vi "Set ParentNode Selected.vi"(7 "Tri-State?":bool=TRUE, 8 "error in (no error)":errorcluster, 9 "Symbol Index":i32, 10 "Tag":string, 11 "TreeControl in":refnum<vi>) -> (0 "error out":errorcluster, 2 "Seted Tags":T1(array[cluster]), 3 "TreeControl out":refnum<vi>)   [LabVIEW 2023, in "DSLV_Tree.lvlib"]
uses:
  DSLV_Tree.lvlib
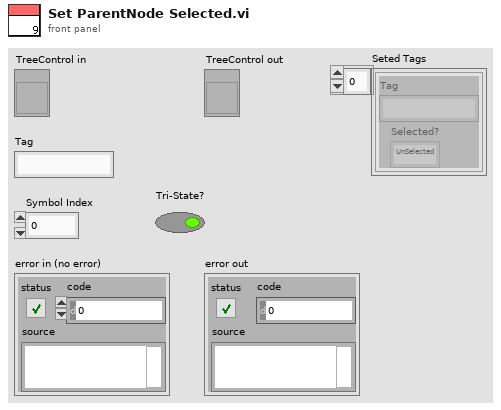
[diagram p1: front panel]
types:
  T1 = cluster{"Tag":string, "Selected?":enum16{"UnSelected", "Selected", "PartSelected"}}[]
  T2 = cluster{"Tag":string, "Selected?":enum16{"UnSelected", "Selected", "PartSelected"}}
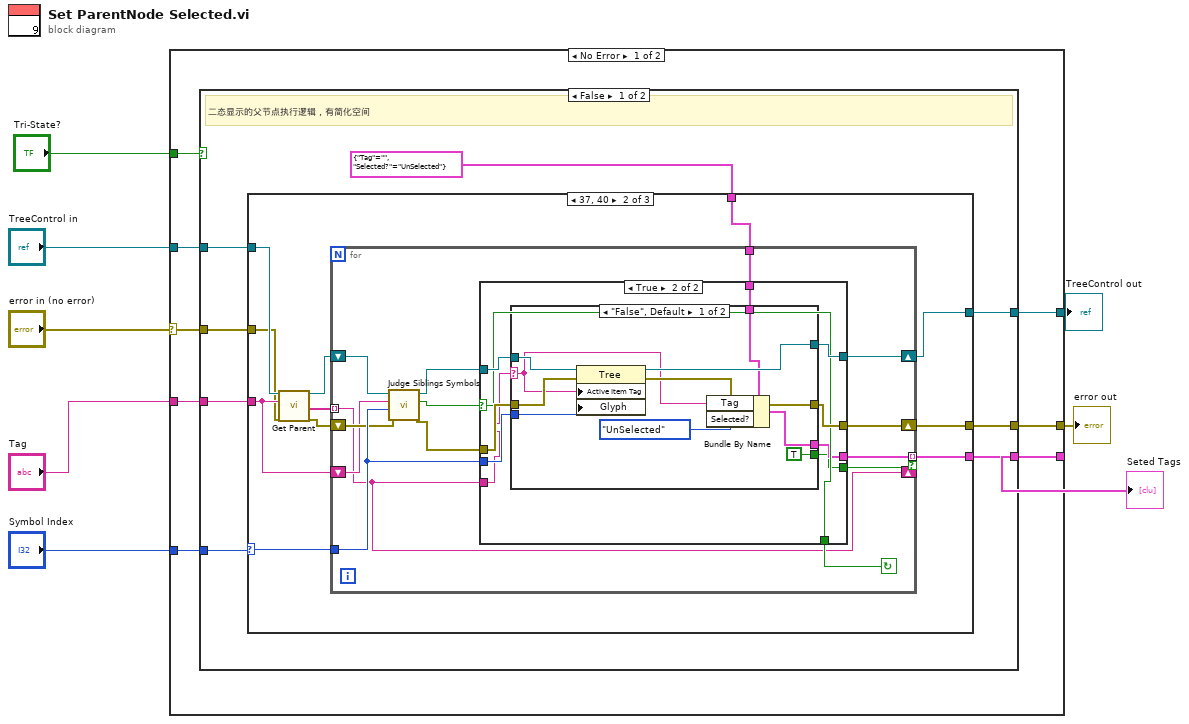
[diagram p0: block diagram]
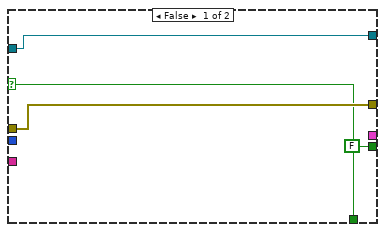
[diagram p3: hidden frame]
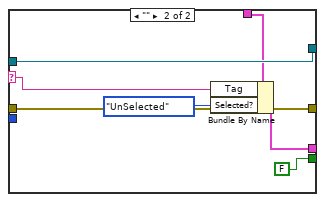
[diagram p4: hidden frame]
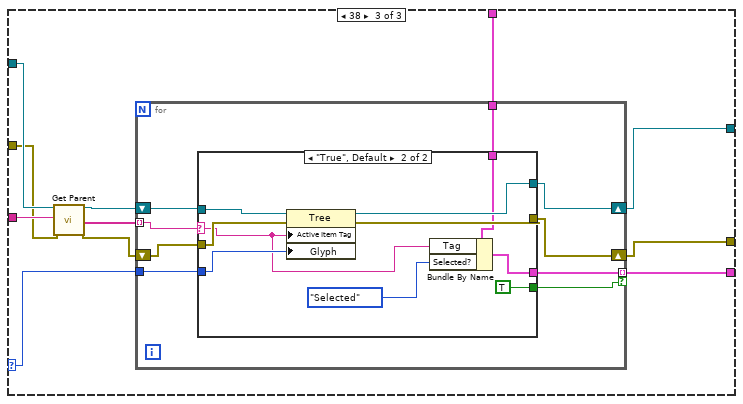
[diagram p5: hidden frame]
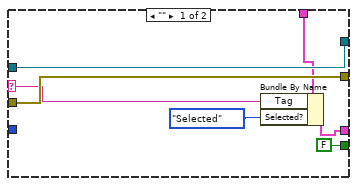
[diagram p6: hidden frame]
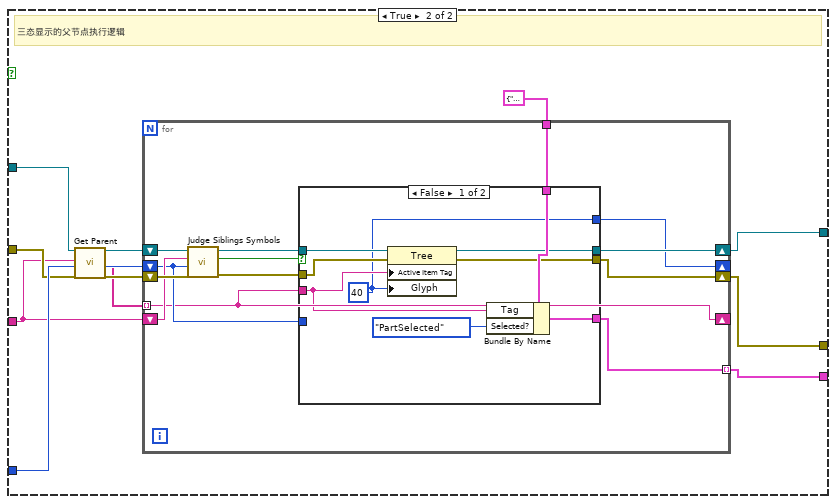
[diagram p7: hidden frame]
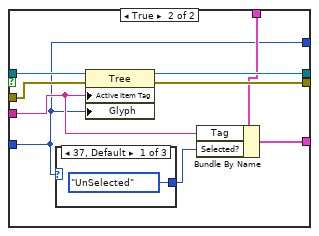
[diagram p8: hidden frame]
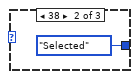
[diagram p9: hidden frame]
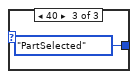
[diagram p10: hidden frame]
diagram:
  n1 = case shown="No Error" "error in (no error)" {
    selector: "error in (no error)" -> [w11 w165]
    tunnel: [w16 w165] -> w8
    tunnel: "Tag" -> [w15 _]
    tunnel: [w14 w166] -> w6
    tunnel: "TreeControl in" -> [w13 w166]
    tunnel: "Symbol Index" -> [w12 _]
    tunnel: [w10 _] -> w2
    tunnel: "Tri-State?" -> [w9 _]
    frame No Error {
      n2 = case shown="False" w9 {
        tunnel: [w24 w120] -> w16
        tunnel: w15 -> [w23 w126]
        tunnel: [w22 w121] -> w14
        tunnel: w13 -> [w21 w129]
        tunnel: w12 -> [w20 w130]
        tunnel: w11 -> [w19 w128]
        tunnel: [w18 w122] -> w10
        frame False {
          # "二态显示的父节点执行逻辑，有简化空间"
          n3 = case shown="37, 40" w20 {
            selector: w20 -> [_ w35 w87]
            tunnel: [w25 w37 w85] -> w24
            tunnel: w23 -> [_ w31 w92]
            tunnel: [w26 w36 w89] -> w22
            tunnel: w19 -> [w25 w30 w86]
            tunnel: w21 -> [w26 w33 w93]
            tunnel: [_ w34 w84] -> w18
            tunnel: T2 {"Tag"="", "Selected?"=enum."UnSelected"} ("Set") -> [_ w27 w83]
            frame -1, Default {
            }
            frame 37, 40 {
              n4 = call "Get Parent.vi"("Tree Reference In"=w33, "Child Tag (Current)"=w31, "error in (no error)"=w30) -> ("Tree Reference Out"=w32:refnum<vi>, "Parents Tags"=w28:string[], "error out"=w29:errorcluster)  [unwired: 13 in, 1 out]
              n5 = for {
                tunnel: w35 -> [w46]
                tunnel: [w45] -> w34 mode=indexing if=w40
                shift-right: [w50] -> w36
                shift-left: w32 -> [w44]
                shift-right: [w51] -> w37
                shift-left: w29 -> [w43]
                tunnel: w28 -> [w38] mode=indexing
                tunnel: w27 -> [w41]
                shift-right: [w38] -> _
                shift-left: w31 -> [w39]
                stop <- w42 continue-if-true
                n6 = call "Judge Siblings Symbols.vi"("error in (no error)"=w43, "Symbol"=w46, "Tag"=w39, "TreeControl in"=w44) -> ("error out"=w48:errorcluster, "The Same?"=w47:bool, "TreeControl out"=w49:refnum<vi>)  [unwired: 5 in]
                n7 = case shown="True" w47 {
                  selector: w47 -> [w53 w59]
                  tunnel: w48 -> [w54 w62]
                  tunnel: w49 -> [w55 w65]
                  tunnel: [w55 w64] -> w50
                  tunnel: [w54 w63] -> w51
                  tunnel: w46 -> [_ w61]
                  tunnel: [_ w57] -> w45
                  tunnel: w38 -> [_ w60]
                  tunnel: [w53 w59] -> w42
                  tunnel: w41 -> [_ w58]
                  tunnel: [FALSE w56] -> w40
                  frame False {
                  }
                  frame True {
                    n8 = case shown="\"False\", Default" w60 {
                      selector: w60 -> [w69 w78]
                      tunnel: w65 -> [w75 w82]
                      tunnel: [w72 w82] -> w64
                      tunnel: w61 -> [w74 _]
                      tunnel: w62 -> [w73 w81]
                      tunnel: [w71 w81] -> w63
                      tunnel: w58 -> [w70 w79]
                      tunnel: [w67 w76] -> w57
                      tunnel: [TRUE FALSE] -> w56
                      frame "False", Default {
                        n9 = property on="Property Node" class="Tree"(reference=w75, error in=w73, "Active Item Tag"=w69, "Glyph"=w74) -> (reference out=w72:refnum<vi>, error out=w71:errorcluster)
                        n10 = Bundle By Name(cluster=w70, "Tag"=w69, "Selected?"=enum16{"UnSelected", "Selected", "PartSelected"}."UnSelected") -> (w67:T2)
                      }
                      frame "" {
                        n11 = Bundle By Name(cluster=w79, "Tag"=w78, "Selected?"=enum16{"UnSelected", "Selected", "PartSelected"}."UnSelected") -> (w76:T2)
                      }
                    }
                  }
                }
              }
            }
            frame 38 {
              n12 = call "Get Parent.vi"("Tree Reference In"=w93, "Child Tag (Current)"=w92, "error in (no error)"=w86) -> ("Tree Reference Out"=w90:refnum<vi>, "Parents Tags"=w91:string[], "error out"=w88:errorcluster)  [unwired: 13 in, 1 out]
              n13 = for {
                tunnel: w91 -> [w102] mode=indexing
                shift-right: [w100] -> w89
                shift-left: w90 -> [w101]
                shift-right: [w97] -> w85
                shift-left: w88 -> [w99]
                tunnel: w87 -> [w98]
                tunnel: [w96] -> w84 mode=indexing if=w95
                tunnel: w83 -> [w94]
                n14 = case shown="\"True\", Default" w102 {
                  selector: w102 -> [w105 w112]
                  tunnel: w101 -> [w108 w119]
                  tunnel: [w108 w118] -> w100
                  tunnel: w99 -> [w109 w117]
                  tunnel: [w109 w116] -> w97
                  tunnel: w98 -> [_ w115]
                  tunnel: [w103 w110] -> w96
                  tunnel: [FALSE TRUE] -> w95
                  tunnel: w94 -> [w106 w113]
                  frame "" {
                    n15 = Bundle By Name(cluster=w106, "Tag"=w105, "Selected?"=enum16{"UnSelected", "Selected", "PartSelected"}."Selected") -> (w103:T2)
                  }
                  frame "True", Default {
                    n16 = property on="Property Node" class="Tree"(reference=w119, error in=w117, "Active Item Tag"=w112, "Glyph"=w115) -> (reference out=w118:refnum<vi>, error out=w116:errorcluster)
                    n17 = Bundle By Name(cluster=w113, "Tag"=w112, "Selected?"=enum16{"UnSelected", "Selected", "PartSelected"}."Selected") -> (w110:T2)
                  }
                }
              }
            }
          }
        }
        frame True {
          # "三态显示的父节点执行逻辑"
          n18 = call "Get Parent.vi"("Tree Reference In"=w129, "Child Tag (Current)"=w126, "error in (no error)"=w128) -> ("Tree Reference Out"=w125:refnum<vi>, "Parents Tags"=w124:string[], "error out"=w127:errorcluster)  [unwired: 13 in, 1 out]
          n19 = for {
            shift-right: [w132] -> _
            shift-left: w126 -> [w139]
            tunnel: w124 -> [w132] mode=indexing
            tunnel: T2 {"Tag"="", "Selected?"=enum."UnSelected"} ("input cluster") -> [w136]
            tunnel: [w135] -> w122 mode=indexing
            shift-right: [w134] -> w121
            shift-left: w125 -> [w142]
            shift-right: [w133] -> w120
            shift-left: w127 -> [w143]
            shift-right: [w131] -> _
            shift-left: w130 -> [w137]
            n20 = call "Judge Siblings Symbols.vi"("error in (no error)"=w143, "Symbol"=w137, "Tag"=w139, "TreeControl in"=w142) -> ("error out"=w138:errorcluster, "The Same?"=w141:bool, "TreeControl out"=w140:refnum<vi>)  [unwired: 5 in]
            n21 = case shown="False" w141 {
              tunnel: w140 -> [w149 w161]
              tunnel: w132 -> [w145 w156]
              tunnel: w138 -> [w147 w160]
              tunnel: w137 -> [_ w153]
              tunnel: [w146 w159] -> w133
              tunnel: [w148 w158] -> w134
              tunnel: w136 -> [w152 w157]
              tunnel: [w151 w155] -> w135
              tunnel: [w144 w153] -> w131
              frame False {
                w144 = 40 ("Active Item:Symbol Index")
                n22 = property on="Property Node" class="Tree"(reference=w149, error in=w147, "Active Item Tag"=w145, "Glyph"=w144) -> (reference out=w148:refnum<vi>, error out=w146:errorcluster)
                n23 = Bundle By Name(cluster=w152, "Tag"=w145, "Selected?"=enum16{"UnSelected", "Selected", "PartSelected"}."PartSelected") -> (w151:T2)
              }
              frame True {
                n24 = case shown="37, Default" w153 {
                  tunnel: [enum16{"UnSelected", "Selected", "PartSelected"}."UnSelected" ("Selected?") enum16{"UnSelected", "Selected", "PartSelected"}."Selected" ("Selected?") enum16{"UnSelected", "Selected", "PartSelected"}."PartSelected" ("Selected?")] -> w154
                  frame 37, Default {
                  }
                  frame 38 {
                  }
                  frame 40 {
                  }
                }
                n25 = property on="Property Node" class="Tree"(reference=w161, error in=w160, "Active Item Tag"=w156, "Glyph"=w153) -> (reference out=w158:refnum<vi>, error out=w159:errorcluster)
                n26 = Bundle By Name(cluster=w157, "Tag"=w156, "Selected?"=w154) -> (w155:T2)
              }
            }
          }
        }
      }
    }
    frame Error {
    }
  }
  "error out" <- w8
  "TreeControl out" <- w6
  "Seted Tags" <- w2
